vi "System Path.vi"(7 "file type":T1(ring), 10 "file name":string) -> (2 "new path":path, 3 "base path":path)   [LabVIEW 2018]
doc: "01.base path：C:\\Inalfa NVH System\\System；Independent of file type\n\n02.new path：it is based on base path"
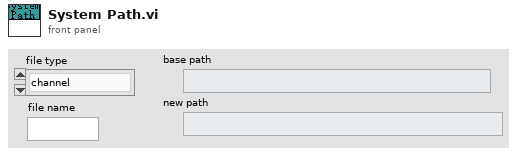
[diagram p1: front panel]
types:
  T1 = enum16{"channel", "data files", "motion", "error table", "part config", "part setup", "tachometer"}
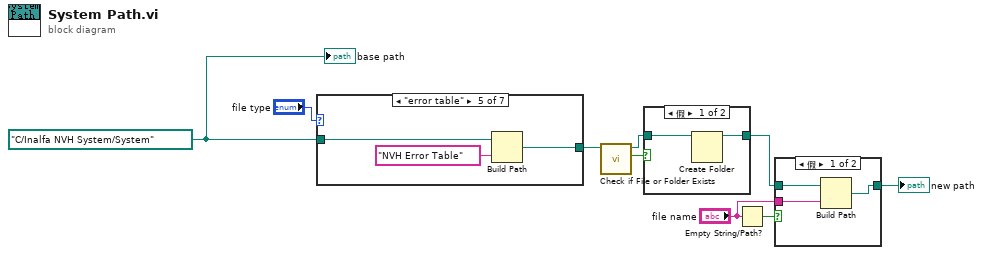
[diagram p0: block diagram]
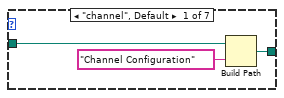
[diagram p2: hidden frame]
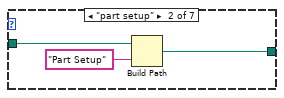
[diagram p3: hidden frame]
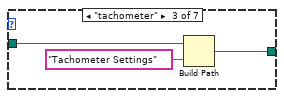
[diagram p4: hidden frame]
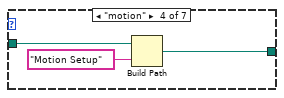
[diagram p5: hidden frame]
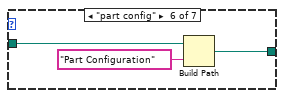
[diagram p6: hidden frame]
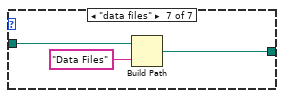
[diagram p7: hidden frame]
diagram:
  w1 = path "C:/Inalfa NVH System/System" ("configuration file path")
  n1 = case shown="\"error table\"" "file type" {
    tunnel: [w10 w13 w17 w20 w23 w26 w29] -> w9
    tunnel: w1 -> [w11 w15 w18 w21 w24 w27 w30]
    frame "channel", Default {
      n2 = Build Path(base path=w11, name or relative path="Channel Configuration" ("名称或相对路径")) -> (appended path=w10:path)
    }
    frame "part setup" {
      n3 = Build Path(base path=w15, name or relative path="Part Setup" ("名称或相对路径")) -> (appended path=w13:path)
    }
    frame "tachometer" {
      n4 = Build Path(base path=w18, name or relative path="Tachometer Settings" ("名称或相对路径")) -> (appended path=w17:path)
    }
    frame "motion" {
      n5 = Build Path(base path=w21, name or relative path="Motion Setup" ("名称或相对路径")) -> (appended path=w20:path)
    }
    frame "error table" {
      n6 = Build Path(base path=w24, name or relative path="NVH Error Table" ("名称或相对路径")) -> (appended path=w23:path)
    }
    frame "part config" {
      n7 = Build Path(base path=w27, name or relative path="Part Configuration" ("名称或相对路径")) -> (appended path=w26:path)
    }
    frame "data files" {
      n8 = Build Path(base path=w30, name or relative path="Data Files" ("名称或相对路径")) -> (appended path=w29:path)
    }
  }
  n9 = call <vilib>:"Check if File or Folder Exists.vi"("path"=w9) -> ("file or folder exists?"=w8:bool, "dup path"=w7:path)  [unwired: 8 in, 1 out]
  n10 = case shown="假" w8 {
    tunnel: w7 -> [w32 w33]
    tunnel: [w31 w33] -> w6
    frame False {
      n11 = Create Folder(path (use dialog)=w32) -> (created path=w31:path)  [unwired: 2 in, 2 out]
    }
    frame True {
    }
  }
  n12 = Empty String/Path?(string/path="file name") -> (empty?=w3:bool)
  n13 = case shown="假" w3 {
    tunnel: w6 -> [w36 w37]
    tunnel: "file name" -> [w35 _]
    tunnel: [w34 w37] -> w5
    frame False {
      n14 = Build Path(base path=w36, name or relative path=w35) -> (appended path=w34:path)
    }
    frame True {
    }
  }
  "new path" <- w5
  "base path" <- w1
